vi "CTRE_PigeonIMU_GetCompass.vi"(8 "error in (no error)":errorcluster, 11 "PigeonIMUDevRef":T2={"DeviceStatus"={"status"=FALSE, "code"=0, "source"=""}, "Device Number"=0, "Type"=352321536, "Device ID"=0, "Handle"=0, "UsageFrame"=0, "Library Path"=path ""} {"Type" items=["CAN"=352321536, "TalonSRX"=33554432]}) -> (0 "error out":errorcluster, 2 "Compass":T1, 3 "PigeonIMUDevRef":T2={"DeviceStatus"={"status"=FALSE, "code"=0, "source"=""}, "Device Number"=0, "Type"=352321536, "Device ID"=0, "Handle"=0, "UsageFrame"=0, "Library Path"=path ""} {"Type" items=["CAN"=352321536, "TalonSRX"=33554432]})   [LabVIEW 2016]
uses:
  <vilib>/Rock Robotics/WPI/ThirdParty/Sensors/Pigeon IMU/CTRE_PigeonIMU_DeviceRef.ctl
  <vilib>/Rock Robotics/WPI/ThirdParty/Sensors/Pigeon IMU/CTRE_PigeonIMU_ConnectionType.ctl
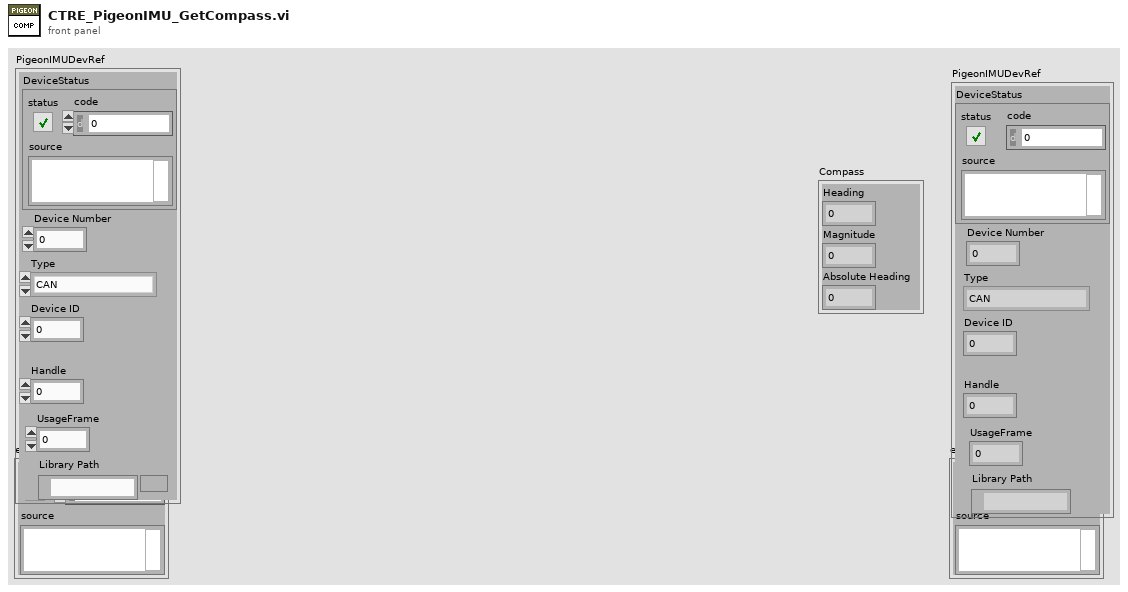
[diagram p1: front panel]
types:
  T1 = cluster{"Heading":dbl, "Magnitude":dbl, "Absolute Heading":dbl}
  T2 = typedef "CTRE_PigeonIMU_DeviceRef.ctl" = cluster{"DeviceStatus":errorcluster, "Device Number":u8, "Type":T3, "Device ID":u32, "Handle":u64, "UsageFrame":u32, "Library Path":path}
  T3 = typedef "CTRE_PigeonIMU_ConnectionType.ctl" = u32
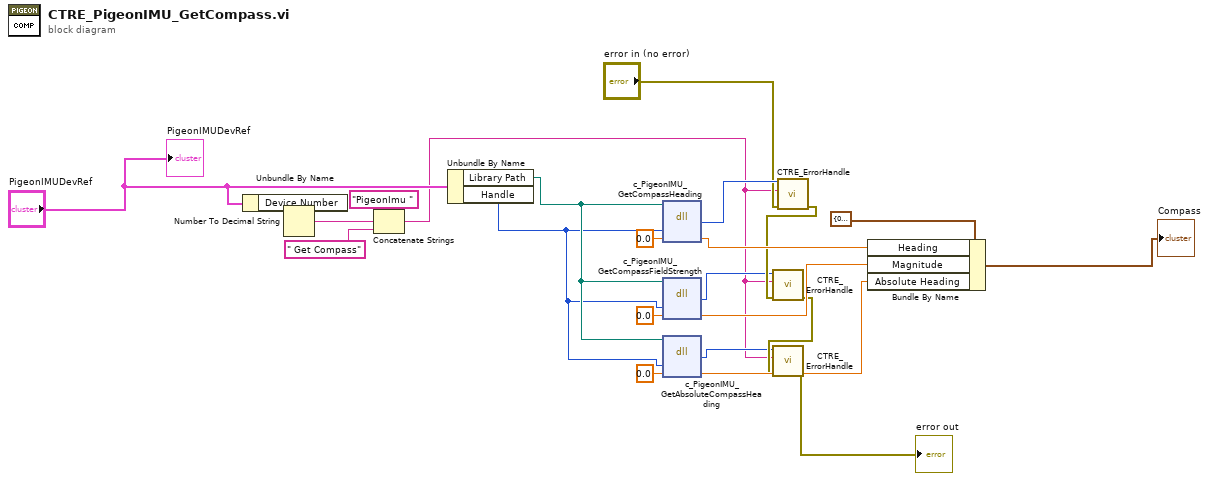
[diagram p0: block diagram]
diagram:
  n1 = Unbundle By Name("PigeonIMUDevRef") -> ("Device Number"=w13:u8)
  n2 = Number To Decimal String(number=w13) -> (decimal integer string=w12:string)  [unwired: 1 in]
  n3 = Concatenate Strings("PigeonImu " ("string"), w12, " Get Compass" ("string")) -> (w1:string)
  n4 = Unbundle By Name("PigeonIMUDevRef") -> ("Library Path"=w17:path, "Handle"=w16:u64)
  n5 = dll-call lib="?" fn="c_PigeonIMU_GetCompassHeading"(path in=w17, "handle"=w16, "value"=0.0) -> ("return type"=w8:i32, "value"=w21:dbl)  [unwired: 3 in, 2 out]
  n6 = dll-call lib="?" fn="c_PigeonIMU_GetCompassFieldStrength"(path in=w17, "handle"=w16, "value"=0.0) -> ("return type"=w3:i32, "value"=w18:dbl)  [unwired: 3 in, 2 out]
  n7 = dll-call lib="?" fn="c_PigeonIMU_GetAbsoluteCompassHeading"(path in=w17, "handle"=w16, "value"=0.0) -> ("return type"=w2:i32, "value"=w15:dbl)  [unwired: 3 in, 2 out]
  n8 = call <vilib>:"CTRE_ErrorHandle.vi"("error in"="error in (no error)", "origin"=w1, "code"=w8) -> ("error out"=w6:errorcluster)  [unwired: 8 in]
  n9 = call <vilib>:"CTRE_ErrorHandle.vi"("error in"=w6, "origin"=w1, "code"=w3) -> ("error out"=w5:errorcluster)  [unwired: 8 in]
  n10 = call <vilib>:"CTRE_ErrorHandle.vi"("error in"=w5, "origin"=w1, "code"=w2) -> ("error out"=→"error out":errorcluster)  [unwired: 8 in]
  n11 = Bundle By Name(cluster=T1 {"Heading"=0.0, "Magnitude"=0.0, "Absolute Heading"=0.0} ("Compass"), "Heading"=w21, "Magnitude"=w18, "Absolute Heading"=w15) -> (→"Compass":T1)
  "PigeonIMUDevRef" <- "PigeonIMUDevRef"
